vi "calculate_min_tolerance_from_string.vi"(8 "error in (no error)":errorcluster, 10 "String":string, 11 "MIN":string) -> (0 "error out":errorcluster, 3 "MIN":dbl)   [LabVIEW 2017]
uses:
  <vilib>/gmath/NI_Gmath.lvlib
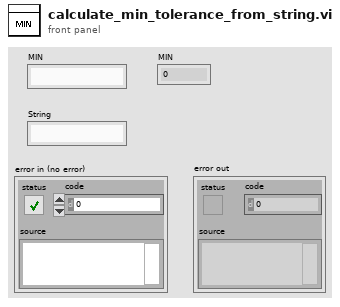
[diagram p1: front panel]
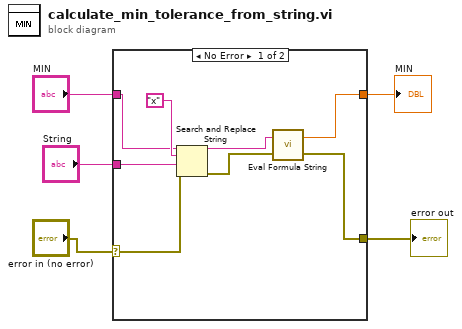
[diagram p0: block diagram]
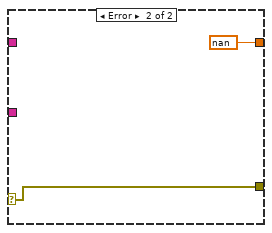
[diagram p2: hidden frame]
diagram:
  n1 = case shown="No Error" "error in (no error)" {
    selector: "error in (no error)" -> [w6 w14]
    tunnel: [w13 nan ("y value")] -> w5
    tunnel: "String" -> [w12 _]
    tunnel: "MIN" -> [w9 _]
    tunnel: [w7 w14] -> w2
    frame No Error {
      n2 = Search and Replace String(input string=w9, search string="x", replace string=w12, error in=w6) -> (result string=w11:string, error out=w8:errorcluster)  [unwired: 4 in, 2 out]
      n3 = call <vilib>:"Eval Formula String.vi"("error in (no error)"=w8, "formula"=w11) -> ("error out"=w7:errorcluster, "y value"=w13:dbl)
    }
    frame Error {
    }
  }
  "MIN" <- w5
  "error out" <- w2
